vi "checkEvent.vi"(0 "standard Visitor":T1, 1 "Event Array":refnum<class "HGF_Event.lvclass">[](array[class]), 3 "Status on event?":bool, 8 "Agent ID":string) -> (13 "Object":refnum<class>, 14 "Event/Null":T2, 16 "timed out":bool, 17 "dup Event Array":refnum<class "HGF_Event.lvclass">[](array[class]), 19 "error out":errorcluster)   [LabVIEW 2009, in "MoAgSy.lvlib" / "MoAgSy_Engine.lvclass"]
uses:
  MoAgSy_Engine.lvclass
  HGF_BaseClasses/HGF_Event/HGF_Event.lvclass
  MoAgSy_StateMachine/MoAgSy_StateMachine.lvsc/Trigger.ctl
  Visitors/MoAgSy_Visitor/MoAgSy_Visitor.lvclass
  MoAgSy_StateMachine/MoAgSy_StateMachine.lvsc
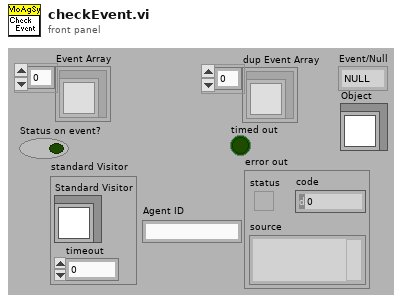
[diagram p1: front panel]
types:
  T1 = cluster{"Standard Visitor":refnum<class "MoAgSy_Visitor.lvclass">, "timeout":dbl}
  T2 = typedef "MoAgSy.lvlib/MoAgSy_StateMachine.lvsc/Trigger.ctl" = enum16{"NULL", "initialized", "Error", "Shutdown", "Event", "Reset", "Ready", "reply", "visitor", "msg", "MoAg", "travel"}
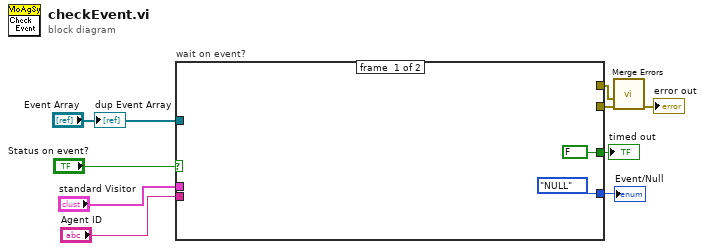
[diagram p0: block diagram]
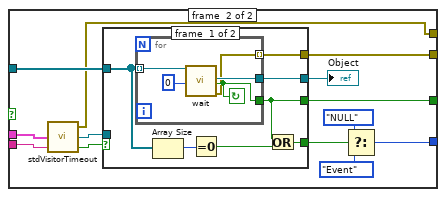
[diagram p2: hidden frame]
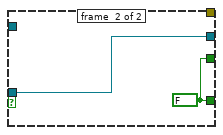
[diagram p3: hidden frame]
diagram:
  n1 = case "wait on event?" shown="True" "Status on event?" {
    tunnel: "Event Array" -> [_ w19]
    tunnel: [Trigger."NULL" ("Trigger") w21] -> w7
    tunnel: [FALSE ("timed out") w20] -> w6
    tunnel: "standard Visitor" -> [_ w17]
    tunnel: "Agent ID" -> [_ w14]
    tunnel: [_ w13] -> w3
    tunnel: [_ w12] -> w1
    frame #0 {
    }
    frame #1 {
      n2 = call "stdVisitorTimeout.vi"("Agent ID"=w14, "standard Visitor"=w17) -> ("stdVisit?"=w15:bool, "dup HGF_NetworkData"=w16:refnum<class "HGF_NetworkVisitor.lvclass">, "error out"=w12:errorcluster)  [unwired: 1 in]
      n3 = case shown="False" w15 {
        tunnel: [w31 w38] -> w22
        tunnel: [w30 w37] -> w20
        tunnel: w19 -> [w29 _]
        tunnel: [w27 w37] -> w18
        tunnel: w16 -> [_ w38]
        tunnel: [w25 _] -> w13
        frame #0 {
          n4 = for {
            tunnel: w29 -> [w36] mode=indexing
            tunnel: [w34] -> w31
            tunnel: [w33] -> w30
            tunnel: [w32] -> w25 mode=indexing
            stop <- w33 continue-if-true
            n5 = call-dynamic "wait.vi"("HGF_Event"=w36, "msTimeout (-1)"=0) -> ("Object"=w34:refnum<class>, "timed out"=w33:bool, "error out"=w32:errorcluster)  [unwired: 2 in, 13 out]
          }
          n6 = Array Size(array=w29) -> (size(s)=w28:i32)
          n7 = Equal To 0?(x=w28) -> (x = 0?=w26:bool)
          n8 = Or(x=w30, y=w26) -> (x .or. y?=w27:bool)
        }
        frame #1 {
          w37 = FALSE
        }
      }
      "Object" <- w22
      n9 = Select(t=Trigger."NULL" ("Trigger"), s=w18, f=Trigger."Event" ("Trigger")) -> (s? t:f=w21:T2)
    }
  }
  "Event/Null" <- w7
  "timed out" <- w6
  n10 = call <vilib>:"Merge Errors.vi"("error array in"=w3, "error in 3 (no error)"=w1) -> ("error out"=→"error out":errorcluster)  [unwired: 5 in]
  "dup Event Array" <- "Event Array"
